vi "XML_slow.vi"(1 "Slow Cluster":T1={"Number of Slow Parameters"=0, "UTC format?"=TRUE, "Sensor Upper bounds"=[85, 1000000, 8000, 8000, 8000, 14000, 99, 33000], "Sensor Lower bounds"=[-40, 0, -8000, -8000, -8000, -14000, 0, -33000], "datanames"=[], "Descriptions"=[]}, 2 "Input String":string) -> (0 "Output String":string)   [LabVIEW 2012]
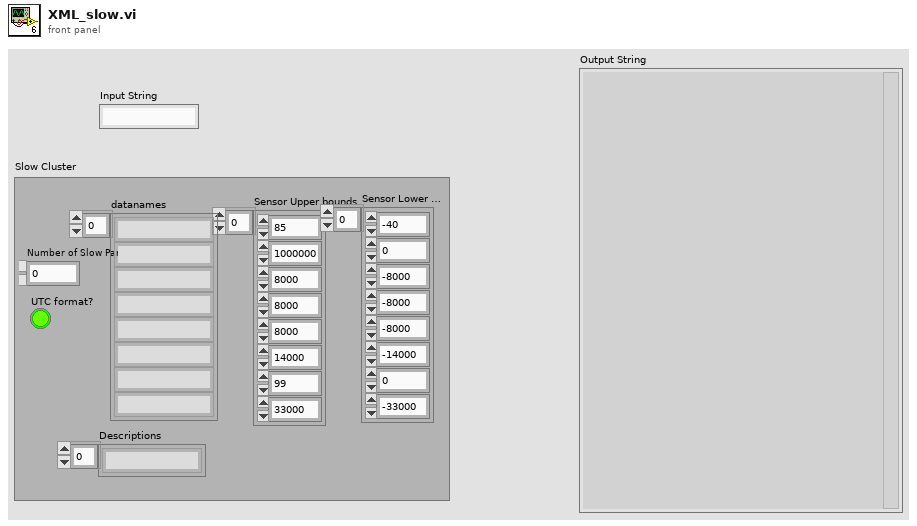
[diagram p1: front panel]
types:
  T1 = cluster{"Number of Slow Parameters":i32, "UTC format?":bool, "Sensor Upper bounds":i32[], "Sensor Lower bounds":i32[], "datanames":string[], "Descriptions":string[]}
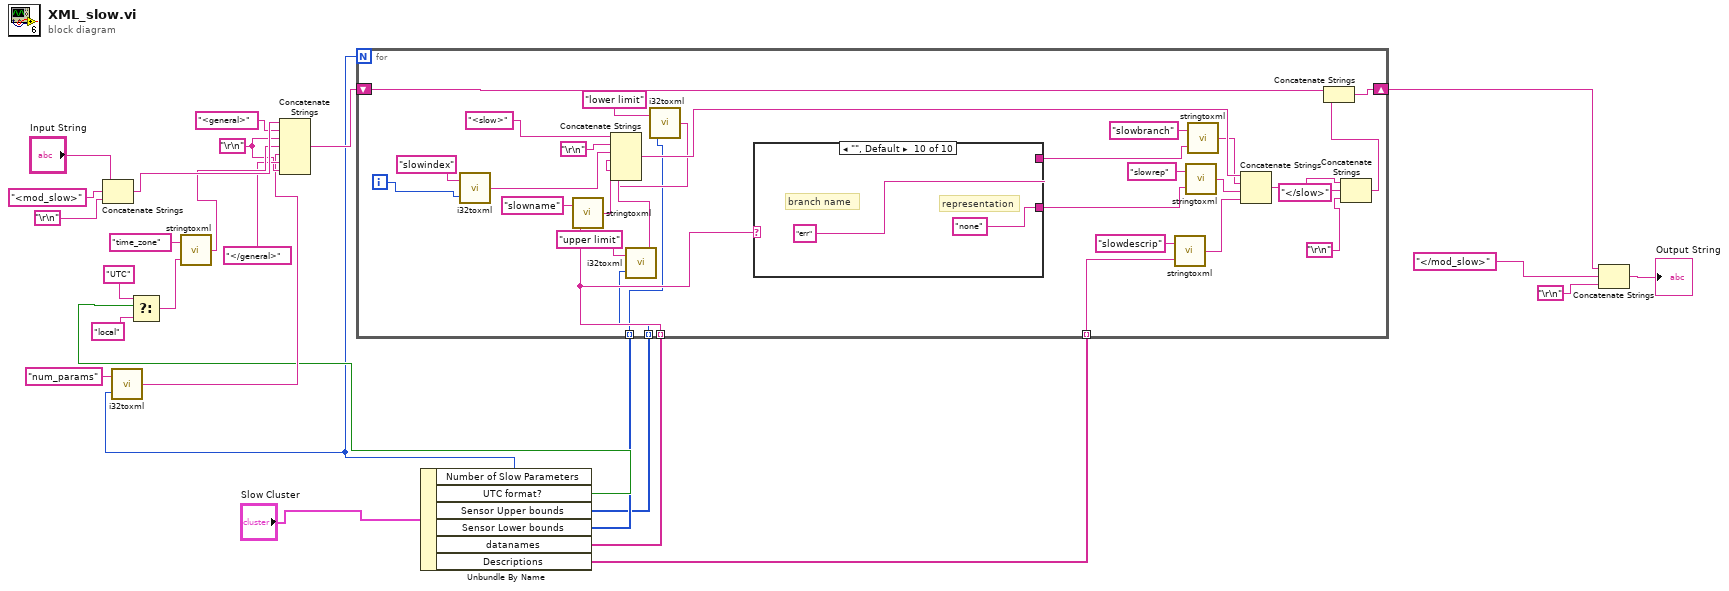
[diagram p0: block diagram]
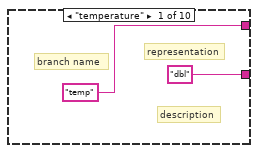
[diagram p2: hidden frame]
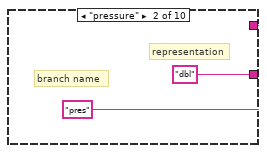
[diagram p3: hidden frame]
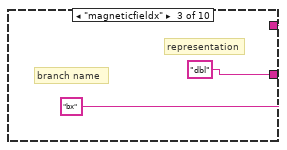
[diagram p4: hidden frame]
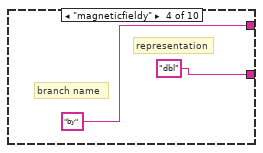
[diagram p5: hidden frame]
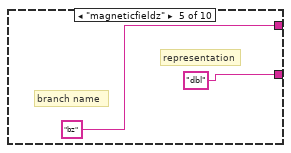
[diagram p6: hidden frame]
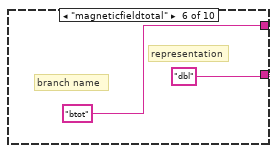
[diagram p7: hidden frame]
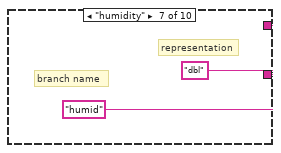
[diagram p8: hidden frame]
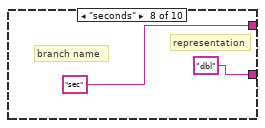
[diagram p9: hidden frame]
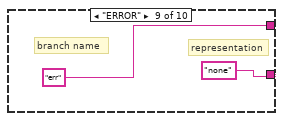
[diagram p10: hidden frame]
diagram:
  w16 = "\r\n"
  n1 = Concatenate Strings("Input String", "<mod_slow>", "\r\n") -> (w20:string)
  n2 = Unbundle By Name("Slow Cluster") -> ("Number of Slow Parameters"=w1:i32, "UTC format?"=w7:bool, "Sensor Upper bounds"=w5:i32[], "Sensor Lower bounds"=w6:i32[], "datanames"=w4:string[], "Descriptions"=w3:string[])
  n3 = call "i32toxml.vi"("variable"=w1, "variable name"="num_params") -> ("xml string"=w12:string)
  n4 = Select(t="UTC" ("XML Tag"), s=w7, f="local") -> (s? t:f=w25:string)
  n5 = call "stringtoxml.vi"("String to write"=w25, "XML Tag"="time_zone") -> ("xml string"=w18:string)
  n6 = Concatenate Strings(w20, "<general>", w16, w18, w12, "</general>" ("string"), w16) -> (w11:string)
  n7 = for {
    N: w1 -> [_]
    shift-right: [w47] -> w9
    shift-left: w11 -> [w56]
    tunnel: w6 -> [w29] mode=indexing
    tunnel: w5 -> [w28] mode=indexing
    tunnel: w4 -> [w30] mode=indexing
    tunnel: w3 -> [w27] mode=indexing
    i -> [w31]
    n8 = call "i32toxml.vi"("variable"=w31, "variable name"="slowindex") -> ("xml string"=w37:string)
    n9 = call "stringtoxml.vi"("String to write"=w30, "XML Tag"="slowname") -> ("xml string"=w46:string)
    n10 = call "i32toxml.vi"("variable"=w28, "variable name"="upper limit") -> ("xml string"=w34:string)
    n11 = call "i32toxml.vi"("variable"=w29, "variable name"="lower limit") -> ("xml string"=w32:string)
    n12 = Concatenate Strings("<slow>" ("string"), "\r\n", w37, w46, w34, w32) -> (w44:string)
    n13 = case shown="\"\", Default" w30 {
      tunnel: ["dbl" ("XML Tag") "dbl" ("XML Tag") "dbl" ("XML Tag") "dbl" ("XML Tag") "dbl" ("XML Tag") "dbl" ("XML Tag") "dbl" ("XML Tag") "dbl" ("XML Tag") "none" ("XML Tag") "none" ("XML Tag")] -> w52
      tunnel: ["temp" "pres" "bx" "by" "bz" "btot" "humid" "sec" "err" "err"] -> w41
      frame "temperature" {
        # "branch name"
        # "description"
        # "representation"
      }
      frame "pressure" {
        # "branch name"
        # "representation"
      }
      frame "magneticfieldx" {
        # "branch name"
        # "representation"
      }
      frame "magneticfieldy" {
        # "branch name"
        # "representation"
      }
      frame "magneticfieldz" {
        # "branch name"
        # "representation"
      }
      frame "magneticfieldtotal" {
        # "branch name"
        # "representation"
      }
      frame "humidity" {
        # "branch name"
        # "representation"
      }
      frame "seconds" {
        # "branch name"
        # "representation"
      }
      frame "ERROR" {
        # "branch name"
        # "representation"
      }
      frame "", Default {
        # "branch name"
        # "representation"
      }
    }
    n14 = call "stringtoxml.vi"("String to write"=w27, "XML Tag"="slowdescrip") -> ("xml string"=w50:string)
    n15 = call "stringtoxml.vi"("String to write"=w52, "XML Tag"="slowrep") -> ("xml string"=w51:string)
    n16 = call "stringtoxml.vi"("String to write"=w41, "XML Tag"="slowbranch") -> ("xml string"=w43:string)
    n17 = Concatenate Strings(w44, w43, w51, w50) -> (w45:string)
    n18 = Concatenate Strings(w45, "</slow>" ("string"), "\r\n") -> (w48:string)
    n19 = Concatenate Strings(w56, w48) -> (w47:string)
  }
  n20 = Concatenate Strings(w9, "</mod_slow>" ("string"), "\r\n") -> (→"Output String":string)
